vi "Round SGL.vi"(11 "SGL":sgl) -> (3 "I32":i32)   [LabVIEW 2020, in "Raster (FPGA).lvlib"]
doc: "Round the SGL to the nearest I32."
uses:
  Raster (FPGA).lvlib
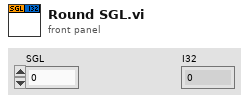
[diagram p1: front panel]
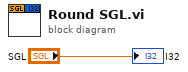
[diagram p0: block diagram]
diagram:
  "I32" <- "SGL"
